vi "Clears Power On Status.vi"(5 "Enable to Query":bool=TRUE, 7 "Enable to Sets":bool=TRUE, 8 "error in":errorcluster, 10 "Clears Power On Status":u16(ring) items=["OFF", "ON"], 11 "VISA resource name":refnum<visa-resource-name>) -> (0 "error out":errorcluster, 2 "Returns the Power On Clear Status":string, 3 "VISA resource name out":refnum<visa-resource-name>)   [LabVIEW 2011, in "DMM4.lvlib"]
uses:
  <instrlib>/DMM4/DMM4.lvlib
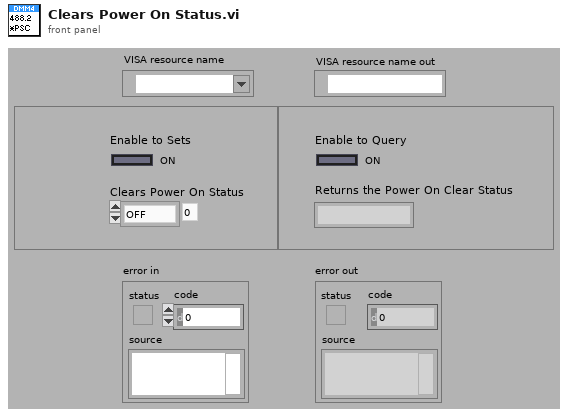
[diagram p1: front panel]
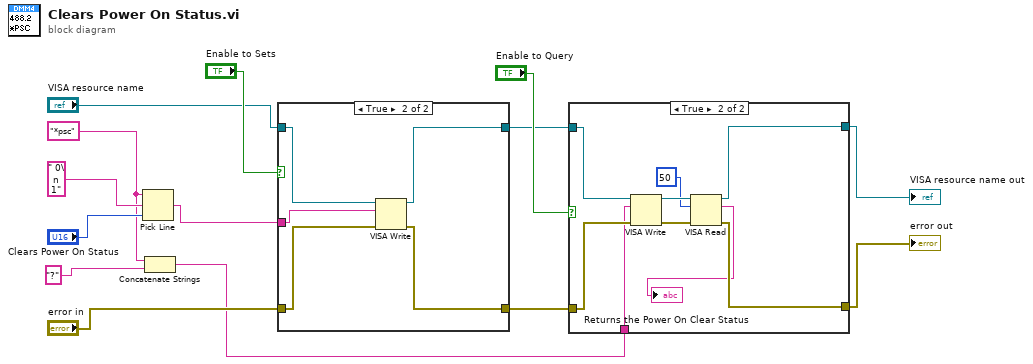
[diagram p0: block diagram]
diagram:
  w12 = "*psc"
  n1 = Pick Line(string ("")=w12, multi-line string=" 0\n 1", line index="Clears Power On Status") -> (output string=w7:string)
  n2 = Concatenate Strings(w12, "?") -> (w3:string)
  n3 = case shown="True" "Enable to Sets" {
    tunnel: "VISA resource name" -> [w16 w21]
    tunnel: "error in" -> [w15 w20]
    tunnel: [w16 w18] -> w5
    tunnel: [w15 w17] -> w4
    tunnel: w7 -> [_ w19]
    frame False {
    }
    frame True {
      n4 = VISA Write(VISA resource name=w21, write buffer=w19, error in (no error)=w20) -> (VISA resource name out=w18:refnum<visa-resource-name>, error out=w17:errorcluster)  [unwired: 1 out]
    }
  }
  n5 = case shown="True" "Enable to Query" {
    tunnel: w5 -> [w23 w29]
    tunnel: w4 -> [w22 w28]
    tunnel: [w23 w26] -> w2
    tunnel: [w22 w25] -> w1
    tunnel: w3 -> [_ w27]
    frame False {
    }
    frame True {
      n6 = VISA Write(VISA resource name=w29, write buffer=w27, error in (no error)=w28) -> (VISA resource name out=w31:refnum<visa-resource-name>, error out=w32:errorcluster)  [unwired: 1 out]
      n7 = VISA Read(VISA resource name=w31, byte count=u32 50, error in (no error)=w32) -> (VISA resource name out=w26:refnum<visa-resource-name>, read buffer=→"Returns the Power On Clear Status":string, error out=w25:errorcluster)  [unwired: 1 out]
    }
  }
  "VISA resource name out" <- w2
  "error out" <- w1
